vi "Update Methods Registration.vi"(8 "error in (no error)":errorcluster, 11 "Server class in":refnum<vi>) -> (0 "error out":errorcluster, 3 "Server class out":refnum<vi>)   [LabVIEW 2019, in "gRPC Template Creation Utility.lvlib"]
uses:
  gRPC Template Creation Utility.lvlib
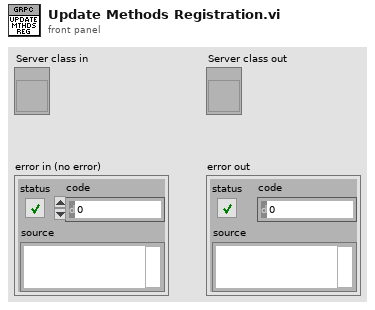
[diagram p1: front panel]
types:
  T1 = typedef "LVPointTypeDef.ctl" = cluster{"Horizontal":i16, "Vertical":i16}
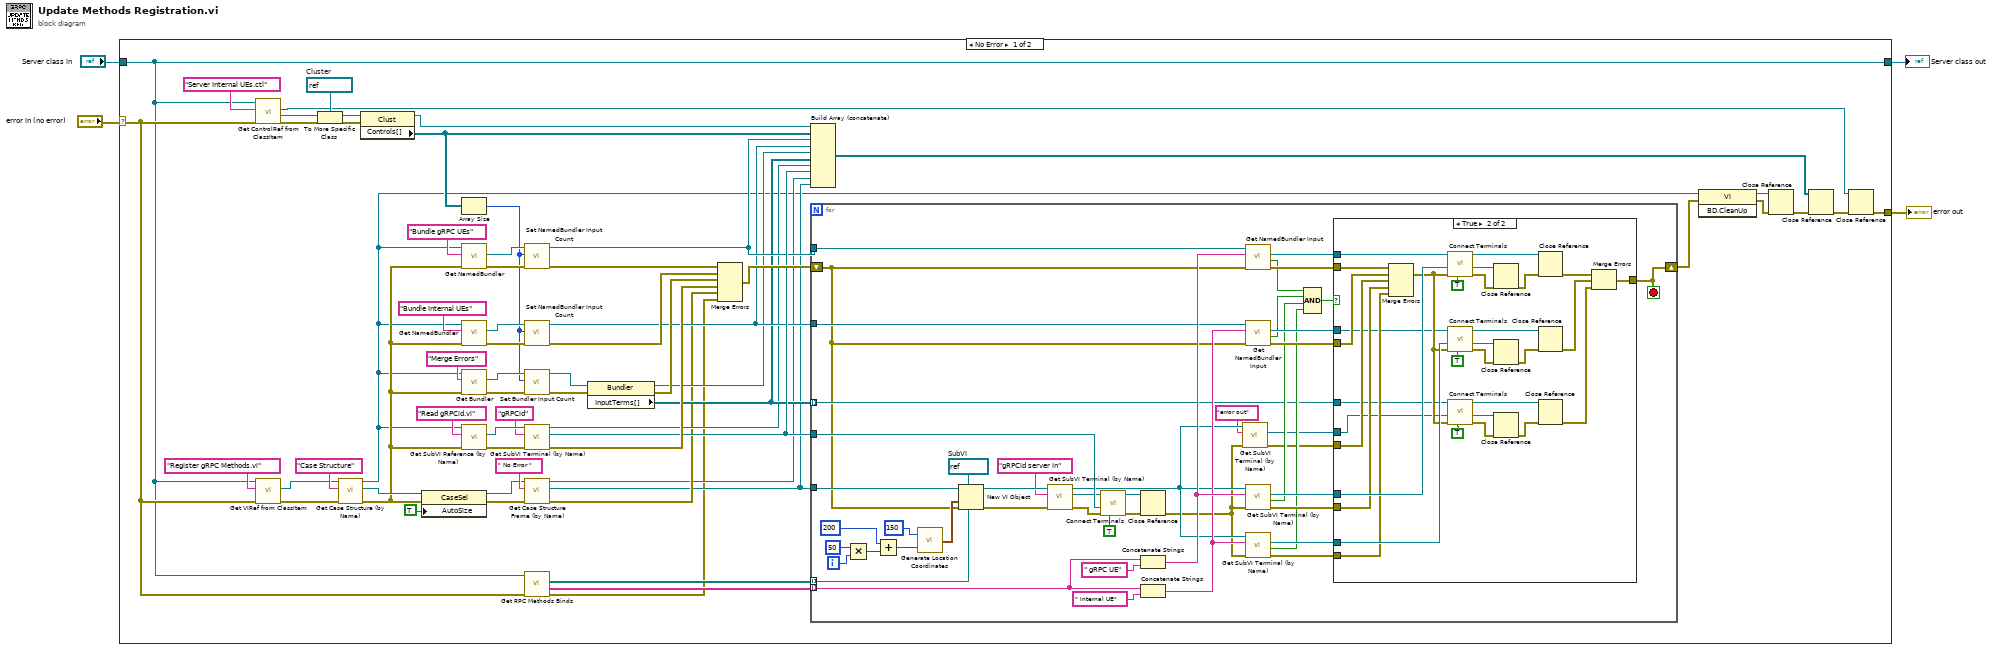
[diagram p0: block diagram]
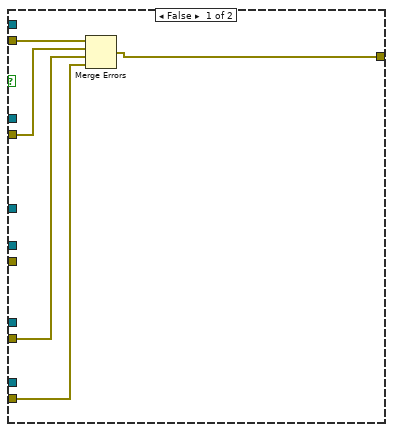
[diagram p2: hidden frame]
diagram:
  n1 = case shown="No Error" "error in (no error)" {
    selector: "error in (no error)" -> [w40 w143]
    tunnel: [w6 w143] -> w4
    tunnel: "Server class in" -> [w39 w144]
    tunnel: [w39 w144] -> w1
    frame No Error {
      w60 = refnum<vi> refnum  # Cluster
      n2 = call "Get ControlRef from ClassItem.vi"("error in (no error)"=w40, "item name"="Server Internal UEs.ctl" ("Item Name"), "class in"=w39) -> ("error out"=w61:errorcluster, "control"=w8:refnum<vi>, "VI ref out"=w5:refnum<vi>)  [unwired: 4 in, 2 out]
      n3 = call "Get VIRef from ClassItem.vi"("error in (no error)"=w40, "item name"="Register gRPC Methods.vi" ("Item Name"), "class in"=w39) -> ("error out"=w56:errorcluster, "vi"=w36:refnum<vi>)  [unwired: 5 in, 2 out]
      n4 = To More Specific Class(target class=w60, reference=w8, error in=w61) -> (specific class reference=w62:refnum<vi>, error out=w63:errorcluster)
      n5 = call "Get Case Structure (by Name).vi"("error in (no error)"=w56, "Case Structure name"="Case Structure" ("y"), "VI ref in"=w36) -> ("error out"=w31:errorcluster, "CaseStructure out"=w46:refnum<vi>, "VI ref out"=w10:refnum<vi>)  [unwired: 5 in, 1 out]
      n6 = property class="Clust"(reference=w62, error in=w63) -> (reference out=w24:refnum<vi>, "Controls[]"=w23:refnum<vi>[])  [unwired: 1 out]
      n7 = property class="CaseSel"(reference=w46, error in=w31, "AutoSize"=TRUE ("AutoSize To Fit Contents?")) -> (reference out=w45:refnum<vi>, error out=w44:errorcluster)
      n8 = Array Size(array=w23) -> (size(s)=w33:i32)
      n9 = call "Get NamedBundler.vi"("error in (no error)"=w31, "Label"="Bundle gRPC UEs" ("name/order"), "Owner VI in"=w10) -> ("error out"=w54:errorcluster, "NamedBundler ref out"=w65:refnum<vi>)  [unwired: 5 in, 2 out]
      n10 = call "Get NamedBundler.vi"("error in (no error)"=w31, "Label"="Bundle Internal UEs" ("name/order"), "Owner VI in"=w10) -> ("error out"=w52:errorcluster, "NamedBundler ref out"=w53:refnum<vi>)  [unwired: 5 in, 2 out]
      n11 = call "Get Bundler.vi"("error in (no error)"=w31, "label"="Merge Errors" ("Label"), "owner vi in"=w10) -> ("error out"=w30:errorcluster, "bundler ref"=w34:refnum<vi>)  [unwired: 5 in, 2 out]
      n12 = call "Get SubVI Reference (by Name).vi"("error in (no error)"=w31, "SubVI Name"="Read gRPCid.vi", "Owner VI in"=w10) -> ("error out"=w49:errorcluster, "SubVI Refnum out"=w50:refnum<vi>)  [unwired: 5 in, 2 out]
      n13 = call "Set NamedBundler Input Count.vi"("error in (no error)"=w54, "Numeric"=w33, "NamedBundler in"=w65) -> ("error out"=w26:errorcluster, "NamedBundler out"=w18:refnum<vi>)  [unwired: 7 in]
      n14 = call "Set NamedBundler Input Count.vi"("error in (no error)"=w52, "Numeric"=w33, "NamedBundler in"=w53) -> ("error out"=w47:errorcluster, "NamedBundler out"=w17:refnum<vi>)  [unwired: 7 in]
      n15 = call "Set Bundler Input Count.vi"("error in (no error)"=w30, "Numeric"=w33, "Bundler in"=w34) -> ("error out"=w29:errorcluster, "Bundler out"=w32:refnum<vi>)  [unwired: 7 in]
      n16 = call "Get SubVI Terminal (by Name).vi"("error in (no error)"=w49, "Terminal name"="gRPCid", "SubVI in"=w50) -> ("error out"=w27:errorcluster, "SubVI Term ref"=w22:refnum<vi>, "SubVI out"=w14:refnum<vi>)  [unwired: 5 in, 1 out]
      n17 = call "Get Case Structure Frame (by Name).vi"("error in (no error)"=w44, "element"=" No Error ", "CaseStructure in"=w45) -> ("error out"=w13:errorcluster, "Frame ref out"=w12:refnum<vi>, "CaseStructure out"=w11:refnum<vi>)  [unwired: 5 in, 1 out]
      n18 = call "Get RPC Methods Binds.vi"("error in (no error)"=w40, "LVClassLibrary in"=w39) -> ("error out"=w9:errorcluster, "RPC Method Binds Names"=w37:string[], "RPC Method Binds Paths"=w38:path[])  [unwired: 6 in, 1 out]
      n19 = property class="Bundler"(reference=w32, error in=w29) -> (reference out=w16:refnum<vi>, error out=w28:errorcluster, "InputTerms[]"=w15:refnum<vi>[])
      n20 = Merge Errors(w26, w47, w28, w27, w13, w9) -> (w25:errorcluster)
      n21 = Build Array (concatenate)(w24, w23, w18, w17, w16, w15, w14, w22, w11, w12) -> (w19:refnum<vi>[])
      n22 = for {
        tunnel: w12 -> [w112]
        tunnel: w18 -> [w111]
        tunnel: w17 -> [w103]
        tunnel: w22 -> [w87]
        tunnel: w38 -> [w76] mode=indexing
        tunnel: w37 -> [w75] mode=indexing
        tunnel: w15 -> [w70] mode=indexing
        shift-right: [w96] -> w21
        shift-left: w25 -> [w68]
        i -> [w85]
        stop <- w96 stop-if-true
        w110 = refnum<vi> refnum  # SubVI
        n23 = Multiply(x=50 ("y"), y=w85) -> (x*y=w83:i32)
        n24 = Add(x=i16 200 ("Horizontal"), y=w83) -> (x+y=w81:i32)
        n25 = call "Generate Location Coordinates.vi"("Vertical"=w81, "Horizontal"=i16 150) -> ("Location out"=w80:T1)
        n26 = New VI Object(vi object class=w110, owner refnum=w112, position/next to=w80, 6:w76, 8:w68) -> (object refnum=w89:refnum<vi>, 0:w90:errorcluster)  [unwired: 3 in]
        n27 = call "Get SubVI Terminal (by Name).vi"("error in (no error)"=w90, "Terminal name"="gRPCid server in", "SubVI in"=w89) -> ("error out"=w77:errorcluster, "SubVI Term ref"=w78:refnum<vi>, "SubVI out"=w74:refnum<vi>)  [unwired: 5 in, 1 out]
        n28 = call "Connect Terminals.vi"("Auto Route? (F)"=TRUE, "Error In"=w77, "Source Terminal"=w87, "Sink Terminal"=w78) -> ("Error Out"=w67:errorcluster)  [unwired: 7 in]
        n29 = Close Reference(reference=w78, error in (no error)=w67) -> (error out=w72:errorcluster)
        n30 = Concatenate Strings(w75, " gRPC UE" ("string")) -> (w106:string)
        n31 = Concatenate Strings(w75, " Internal UE" ("string")) -> (w104:string)
        n32 = call "Get SubVI Terminal (by Name).vi"("error in (no error)"=w72, "Terminal name"="error out", "SubVI in"=w74) -> ("error out"=w71:errorcluster, "SubVI Term ref"=w69:refnum<vi>)  [unwired: 5 in, 2 out]
        n33 = call "Get NamedBundler Input.vi"("error in (no error)"=w68, "Input name"=w106, "NamedBundler ref in"=w111) -> ("error out"=w100:errorcluster, "Found?"=w95:bool, "Input Term ref"=w109:refnum<vi>)  [unwired: 5 in, 1 out]
        n34 = call "Get NamedBundler Input.vi"("error in (no error)"=w68, "Input name"=w104, "NamedBundler ref in"=w103) -> ("error out"=w98:errorcluster, "Found?"=w94:bool, "Input Term ref"=w102:refnum<vi>)  [unwired: 5 in, 1 out]
        n35 = call "Get SubVI Terminal (by Name).vi"("error in (no error)"=w72, "Terminal name"=w106, "SubVI in"=w74) -> ("error out"=w99:errorcluster, "Found?"=w93:bool, "SubVI Term ref"=w108:refnum<vi>)  [unwired: 5 in, 1 out]
        n36 = call "Get SubVI Terminal (by Name).vi"("error in (no error)"=w72, "Terminal name"=w104, "SubVI in"=w74) -> ("error out"=w97:errorcluster, "Found?"=w92:bool, "SubVI Term ref"=w101:refnum<vi>)  [unwired: 5 in, 1 out]
        n37 = Compound Arithmetic op=AND(w95, w94, w93, w92) -> (w91:bool)
        n38 = case shown="True" w91 {
          tunnel: w109 -> [_ w121]
          tunnel: w108 -> [_ w139]
          tunnel: w102 -> [_ w124]
          tunnel: w101 -> [_ w138]
          tunnel: w100 -> [w117 w137]
          tunnel: w99 -> [w114 w134]
          tunnel: w98 -> [w115 w136]
          tunnel: w97 -> [w113 w133]
          tunnel: [w116 w142] -> w96
          tunnel: w71 -> [_ w135]
          tunnel: w70 -> [_ w129]
          tunnel: w69 -> [_ w127]
          frame False {
            n39 = Merge Errors(w117, w115, w114, w113) -> (w116:errorcluster)
          }
          frame True {
            n40 = Merge Errors(w137, w136, w135, w134, w133) -> (w131:errorcluster)
            n41 = call "Connect Terminals.vi"("Auto Route? (F)"=TRUE, "Error In"=w131, "Source Terminal"=w139, "Sink Terminal"=w121) -> ("Error Out"=w119:errorcluster)  [unwired: 7 in]
            n42 = call "Connect Terminals.vi"("Auto Route? (F)"=TRUE, "Error In"=w131, "Source Terminal"=w138, "Sink Terminal"=w124) -> ("Error Out"=w125:errorcluster)  [unwired: 7 in]
            n43 = call "Connect Terminals.vi"("Auto Route? (F)"=TRUE, "Error In"=w131, "Source Terminal"=w127, "Sink Terminal"=w129) -> ("Error Out"=w128:errorcluster)  [unwired: 7 in]
            n44 = Close Reference(reference=w139, error in (no error)=w119) -> (error out=w120:errorcluster)
            n45 = Close Reference(reference=w138, error in (no error)=w125) -> (error out=w123:errorcluster)
            n46 = Close Reference(reference=w127, error in (no error)=w128) -> (error out=w130:errorcluster)
            n47 = Close Reference(reference=w121, error in (no error)=w120) -> (error out=w118:errorcluster)
            n48 = Close Reference(reference=w124, error in (no error)=w123) -> (error out=w122:errorcluster)
            n49 = Close Reference(reference=w129, error in (no error)=w130) -> (error out=w126:errorcluster)
            n50 = Merge Errors(w118, w122, w126) -> (w142:errorcluster)
          }
        }
      }
      n51 = invoke class="VI" method="BD.CleanUp"(reference=w10, error in=w21) -> (reference out=w42:refnum<vi>, error out=w41:errorcluster)  [unwired: 1 in, 1 out]
      n52 = Close Reference(reference=w42, error in (no error)=w41) -> (error out=w20:errorcluster)
      n53 = Close Reference(reference=w19, error in (no error)=w20) -> (error out=w7:errorcluster)
      n54 = Close Reference(reference=w5, error in (no error)=w7) -> (error out=w6:errorcluster)
    }
    frame Error {
    }
  }
  "error out" <- w4
  "Server class out" <- w1
